vi "synnax writer open Single.vi"(4 "enable_auto_commit (T)":bool=TRUE, 5 "err_on_unauthorized (F)":bool, 6 "auto_index (F)":bool, 7 "start (now)":timestamp, 8 "error in":errorcluster, 9 "authorities (255 for all channels)":u8[](array[numeric]), 10 "channel in":u32, 11 "client in":u64) -> (0 "error out":errorcluster, 2 "channel out":u32, 3 "writer out":u64)   [LabVIEW 2026, in "synnax_clib.lvlib"]
doc: "SYNNAX_EXPORT int32_t synnax_writer_open(\n SynnaxClient client,\n int64_t start,\n const uint32_t *channels,\n uint64_t channel_count,\n int32_t mode,\n int32_t enable_auto_commit,\n SynnaxWriter *out_writer,\n SynnaxError err\n);"
uses:
  synnax_clib.lvlib
  typedefs/writer_mode.ctl
  Timestamp Conversion Single.vi
  synnax_clib.dll
panel:
  out "client out":u64
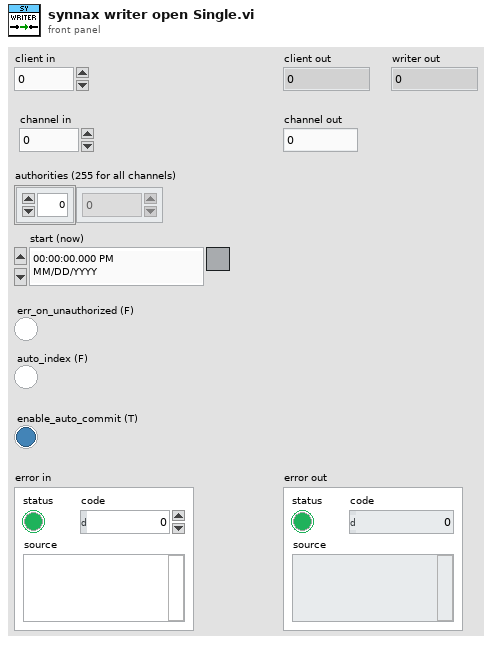
[diagram p1: front panel]
types:
  T1 = typedef "synnax_clib.lvlib/writer_mode.ctl" = enum16{"PERSIST & STREAM", "PERSIST", "STREAM"}
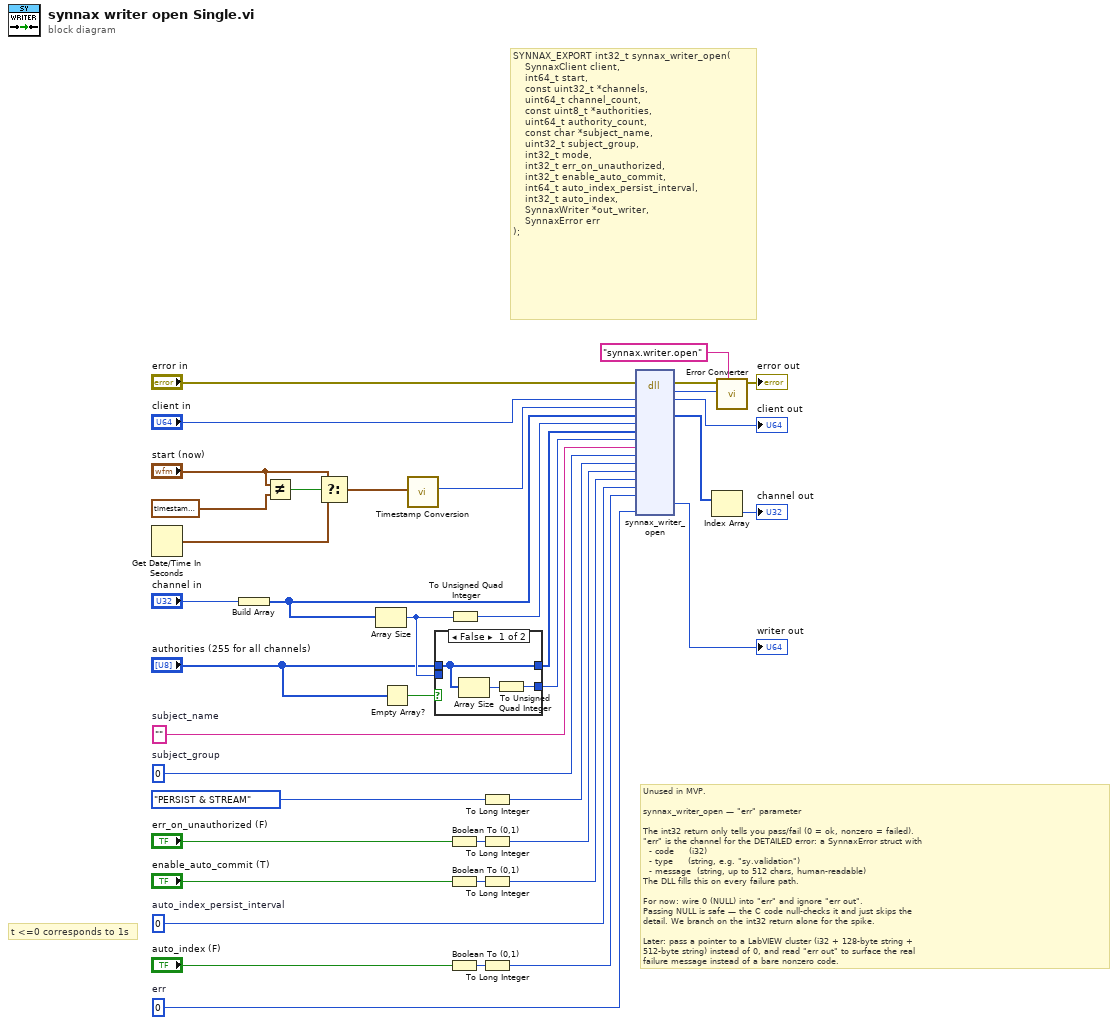
[diagram p0: block diagram]
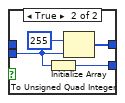
[diagram p2: hidden frame]
diagram:
  w20 = i64 0  # auto_index_persist_interval
  w24 = u32 0  # subject_group
  w25 = ""  # subject_name
  w34 = u64 0  # err
  # "t <=0 corresponds to 1s"
  # "Unused in MVP.\n\nsynnax_writer_open — \"err\" parameter\n\nThe int32 return only tells you pass/fail (0 = ok, nonzero = failed).\n\"err\" is the channel for the DETAILED error: a SynnaxError struct with\n  - code     (i32)\n  - type     (string, e.g. \"sy.validation\")\n  - message  (string, up to 512 chars, human-readable)\nThe DLL fills this on every failure path.\n\nFor now: wire 0 (NULL) into \"err\" and ignore \"err out\".\nPassing NULL is safe — the C code null-checks it and just skips the\ndetail. We branch on the int32 return alone for the spike.\n\nLater: pass a pointer to a LabVIEW cluster (i32 + 128-byte string +\n512-byte string) instead of 0, and read \"err out\" to surface the real\nfailure message instead of a bare nonzero code."
  # "SYNNAX_EXPORT int32_t synnax_writer_open(\n    SynnaxClient client,\n    int64_t start,\n    const uint32_t *channels,\n    uint64_t channel_count,\n    const uint8_t *authorities,\n    uint64_t authority_count,\n    const char *subject_name,\n    uint32_t subject_group,\n    int32_t mode,\n    int32_t err_on_unauthorized,\n    int32_t enable_auto_commit,\n    int64_t auto_index_persist_interval,\n    int32_t auto_index,\n    SynnaxWriter *out_writer,\n    SynnaxError err\n);"
  n1 = Get Date/Time In Seconds() -> (seconds since 1Jan1904=w7:timestamp)
  n2 = Build Array("channel in") -> (w3:u32[])
  n3 = Not Equal?(x="start (now)", y=timestamp timestamp(0 s since 1904-01-01)) -> (x != y?=w10:bool)
  n4 = Select(t="start (now)", s=w10, f=w7) -> (s? t:f=w6:timestamp)
  n5 = Array Size(array=w3) -> (size(s)=w15:i32)
  n6 = Empty Array?(array="authorities (255 for all channels)") -> (empty?=w13:bool)
  n7 = call-poly "Timestamp Conversion.vi"("timestamp"=w6) -> ("timestamp (ns)"=w5:i64)  [unwired: 9 in]
  n8 = case shown="False" w13 {
    tunnel: [w41 w46] -> w16
    tunnel: w15 -> [_ w44]
    tunnel: "authorities (255 for all channels)" -> [w41 _]
    tunnel: [w40 w43] -> w11
    frame False {
      n9 = Array Size(array=w41) -> (size(s)=w42:i32)
      n10 = To Unsigned Quad Integer(1:w42) -> (0:w40:u64)
    }
    frame True {
      n11 = To Unsigned Quad Integer(1:w44) -> (0:w43:u64)
      n12 = Initialize Array(u8 255, w44) -> (w46:u8[])
    }
  }
  n13 = Boolean To (0,1)(Boolean="err_on_unauthorized (F)") -> (0, 1=w22:i16)
  n14 = Boolean To (0,1)(Boolean="enable_auto_commit (T)") -> (0, 1=w35:i16)
  n15 = Boolean To (0,1)(Boolean="auto_index (F)") -> (0, 1=w18:i16)
  n16 = To Unsigned Quad Integer(1:w15) -> (0:w14:u64)
  n17 = To Long Integer(number=writer_mode."PERSIST & STREAM") -> (32bit integer=w26:i32)
  n18 = To Long Integer(number=w22) -> (32bit integer=w21:i32)
  n19 = To Long Integer(number=w35) -> (32bit integer=w33:i32)
  n20 = To Long Integer(number=w18) -> (32bit integer=w17:i32)
  n21 = dll-call lib="C/synnax/client/labview/synnax_clib.*" fn="synnax_writer_open"(error in="error in", "client"="client in", "start"=w5, "channels"=w3, "channel_count"=w14, "authorities"=w16, "authority_count"=w11, "subject_name"=w25, "subject_group"=w24, "mode"=w26, "err_on_unauthorized"=w21, "enable_auto_commit"=w33, "auto_index_persist_interval"=w20, "auto_index"=w17, "err"=w34) -> (error out=w32:errorcluster, "return type"=w31:i32, "client"=→"client out":u64, "channels"=w2:u32[], "out_writer"=→"writer out":u64)  [unwired: 15 in, 1 out]
  n22 = Index Array(array=w2) -> (element=→"channel out":u32)  [unwired: 1 in]
  n23 = call "Error Converter.vi"("source"="synnax.writer.open", "error code"=w31, "error in (no error)"=w32) -> ("error out"=→"error out":errorcluster)  [unwired: 8 in]
